vi "Zadanie11.vi"() -> ()   [LabVIEW 2020]
doc: "Project of sound reciving program, made by Rados³aw Bielak."
uses:
  <vilib>/sound2/lvsound2.llb/Sound Data Format.ctl
  Ctr4.ctl
  Ctr3.ctl
  datacons.ctl
  <vilib>/sound2/lvsound2.llb/Sound Input Task ID.ctl
  <vilib>/sound2/lvsound2.llb/Sampling Mode.ctl
  <vilib>/sound2/lvsound2.llb/Sound Input Read (DBL).vi
  <vilib>/sound2/lvsound2.llb/Sound File Write Open.vi
  <vilib>/sound2/lvsound2.llb/Sound File Write (DBL).vi
  <vilib>/measure/maspectr.llb/FFT Power Spectrum and PSD for N Chan.vi
  <vilib>/measure/NI_MAPro.lvlib
panel:
  in  "File Path":path
  in  "Sound Format":T1={"sample rate (S/s)"=22050.0, "number of channels"=2, "bits per sample"=16}
  in  "Sample Rate":i32=10000
  in  "Exit":bool
  in  "Play":bool
  in  "Tab Control":enum32{"Time Signal", "Power Spectrum"}(tab)
  out "Time Signal":waveform(dbl)[](graph)
  out "Power Spectrum":cluster{"f0":dbl, "df":dbl, "magnitude":dbl[]}[](graph)
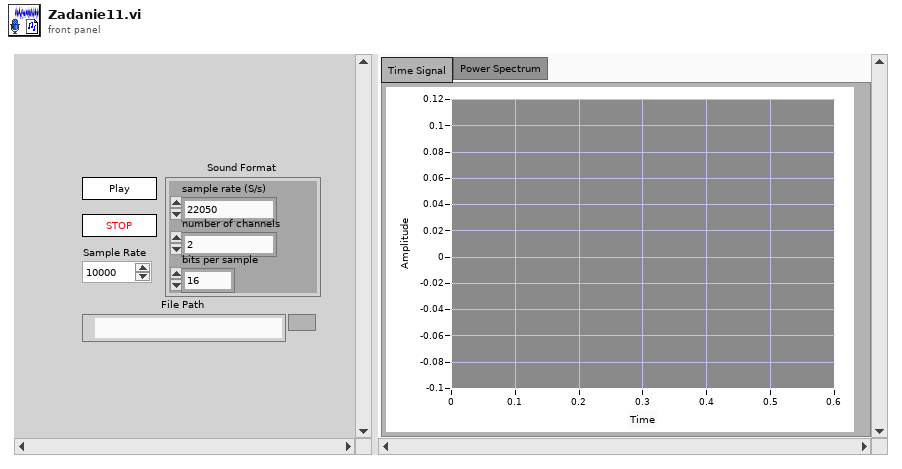
[diagram p1: front panel]
types:
  T1 = typedef "Sound Data Format.ctl" = cluster{"sample rate (S/s)":dbl, "number of channels":i32, "bits per sample":i32}
  T2 = typedef "Ctr4.ctl" = cluster{"Enum":T3, "data":variant}
  T3 = typedef "Ctr3.ctl" = enum16{"time", "spectrum"}
  T4 = typedef "datacons.ctl" = cluster{"Play":bool, "number of samples/ch":i32, "sound format":T1}
  T5 = typedef "Sound File Refnum.ctl" = refnum<file>
  T6 = typedef "Sound Input Task ID.ctl" = u32
  T7 = typedef "Sampling Mode.ctl" = i32
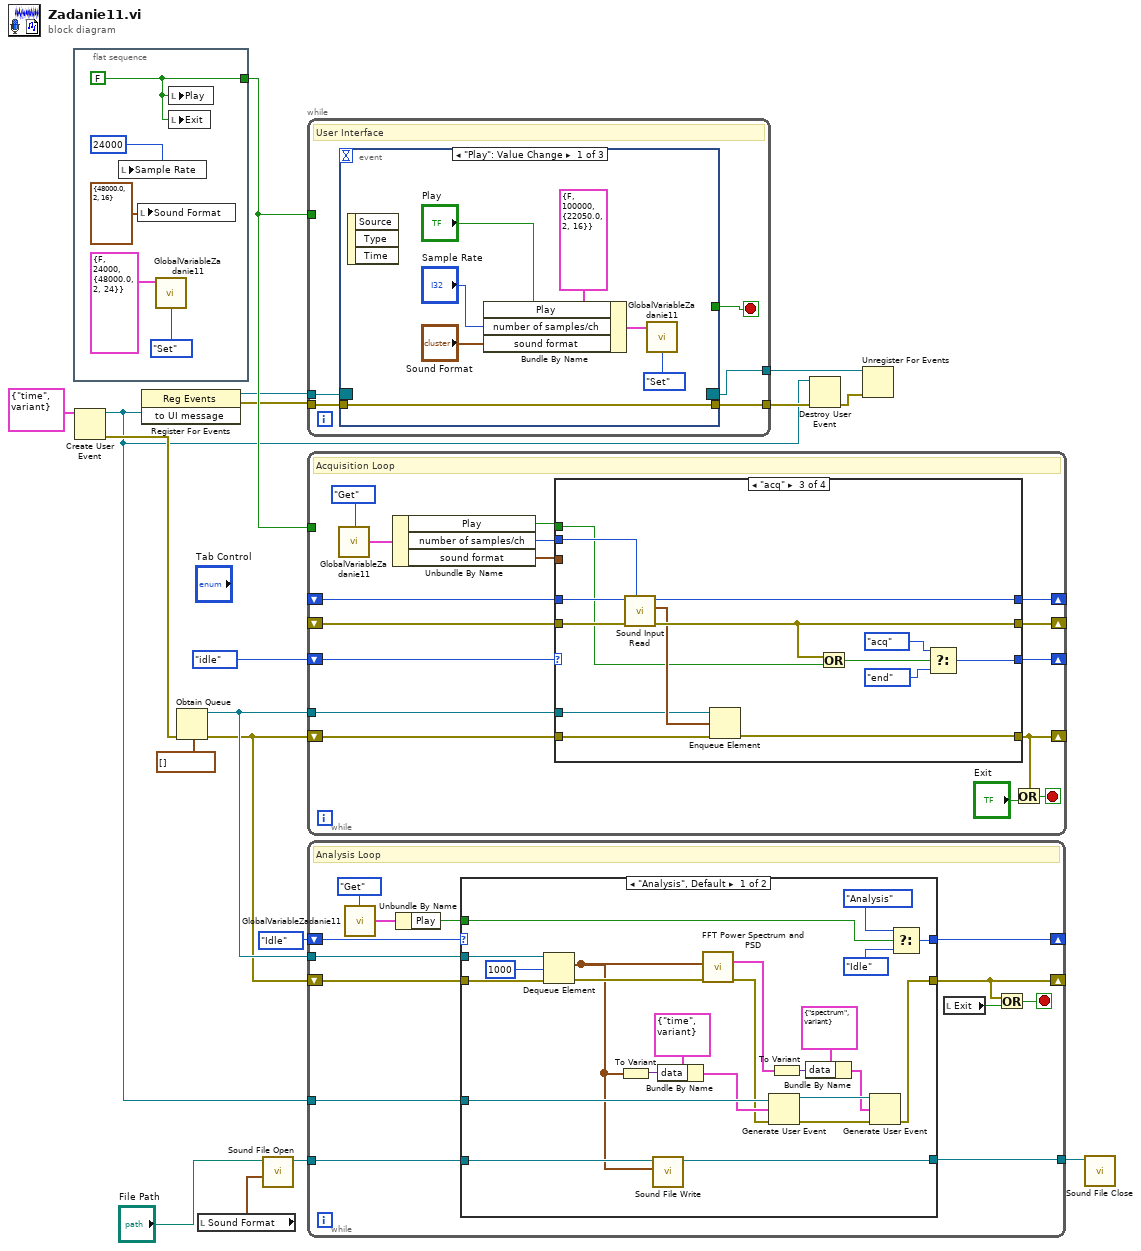
[diagram p0: block diagram]
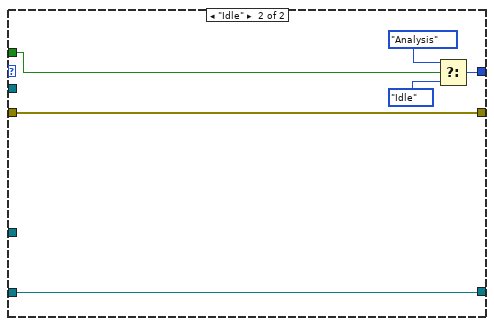
[diagram p2: hidden frame]
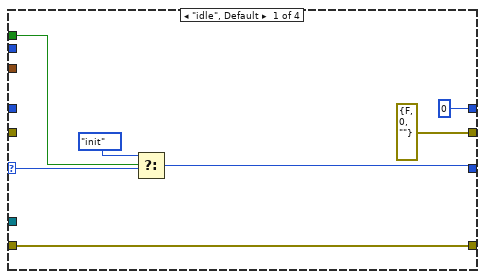
[diagram p3: hidden frame]
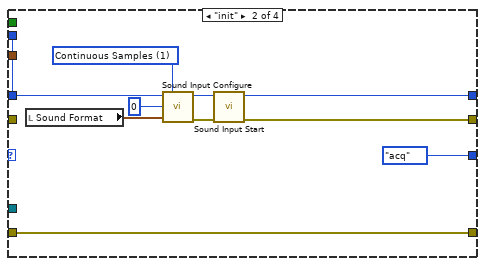
[diagram p4: hidden frame]
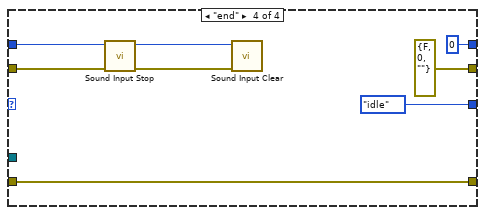
[diagram p5: hidden frame]
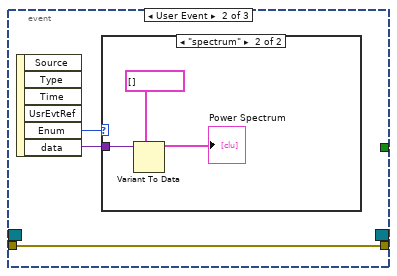
[diagram p6: hidden frame]
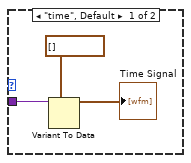
[diagram p7: hidden frame]
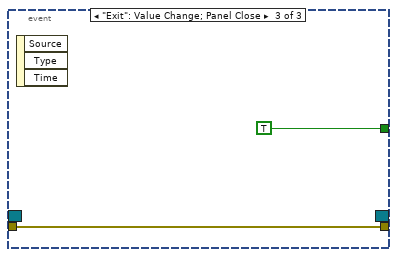
[diagram p8: hidden frame]
diagram:
  n1 = flat-sequence {
    tunnel: [w21] -> w18
    frame #0 {
      w21 = FALSE
      n2 = local write "Sample Rate"(24000) -> ()
      n3 = local write "Sound Format"(T1 {"sample rate (S/s)"=48000.0, "number of channels"=2, "bits per sample"=16} ("sound format")) -> ()
      n4 = call "GlobalVariableZadanie11.vi"("Action"=enum16{"Set", "Get"}."Set", "input"=T4 {"Play"=FALSE, "number of samples/ch"=24000, "sound format"={"sample rate (S/s)"=48000.0, "number of channels"=2, "bits per sample"=24}} ("cluster")) -> ()  [unwired: 9 in, 1 out]
      n5 = local write "Play"(w21) -> ()
      n6 = local write "Exit"(w21) -> ()
    }
  }
  n7 = Create User Event(user event datatype=T2 {"Enum"=enum."time", "data"=variant} ("to UI message")) -> (user event=w5:refnum<user-event>, error out=w13:errorcluster)  [unwired: 1 in]
  n8 = register-events(w5) -> (reference out=w9:refnum<event-registration>, error out=w8:errorcluster)  [unwired: 2 in]
  n9 = Obtain Queue(element data type=waveform(dbl)[] [] ("data"), error in (no error)=w13) -> (queue out=w16:refnum<queue>, error out=w10:errorcluster)  [unwired: 3 in, 1 out]
  n10 = local read "Sound Format"() -> (w4:T1)
  n11 = call-poly <vilib>:"Sound File Open.vi"("sound format"=w4, "path"="File Path") -> ("sound file refnum"=w3:T5)  [unwired: 8 in, 1 out]
  n12 = while "User Interface" {
    tunnel: w18 -> [_]
    tunnel: [w27] -> w12
    tunnel: w9 -> [w26]
    tunnel: w8 -> [w25]
    tunnel: [w24] -> w7
    stop <- w28 stop-if-true
    # "User Interface"
    n13 = event shown="[0] \"Play\": Value Change" {
      selector: w26 -> [_ _ _]
      dyn-events: [_ _ _] -> w27
      timeout: _ -> [_ _ _]
      tunnel: [_ _ TRUE] -> w28
      tunnel: w25 -> [w29 w36 w45]
      tunnel: [w29 w36 w45] -> w24
      event "Play": Value Change {
        n14 = event-data() -> ()  [unwired: 1 in, 3 out]
        n15 = Bundle By Name(cluster=T4 {"Play"=FALSE, "number of samples/ch"=100000, "sound format"={"sample rate (S/s)"=22050.0, "number of channels"=2, "bits per sample"=16}}, "Play"="Play", "number of samples/ch"="Sample Rate", "sound format"="Sound Format") -> (w31:T4)
        n16 = call "GlobalVariableZadanie11.vi"("Action"=enum16{"Set", "Get"}."Set", "input"=w31) -> ()  [unwired: 9 in, 1 out]
      }
      event User Event {
        n17 = event-data() -> ("Enum"=w38:T3, "data"=w37:variant)  [unwired: 1 in, 4 out]
        n18 = case shown="\"spectrum\"" w38 {
          tunnel: w37 -> [w41 w44]
          frame "time", Default {
            n19 = Variant To Data(type=waveform(dbl)[] [] ("element"), Variant=w41) -> (data=→"Time Signal":waveform(dbl)[])  [unwired: 1 in, 1 out]
          }
          frame "spectrum" {
            n20 = Variant To Data(type=cluster{"f0":dbl, "df":dbl, "magnitude":dbl[]}[] [] ("Power Spectrum / PSD"), Variant=w44) -> (data=→"Power Spectrum":cluster{"f0":dbl, "df":dbl, "magnitude":dbl[]}[])  [unwired: 1 in, 1 out]
          }
        }
      }
      event "Exit": Value Change; Panel Close {
        n21 = event-data() -> ()  [unwired: 1 in, 3 out]
      }
    }
  }
  n22 = while {
    tunnel: [w63] -> _
    tunnel: w18 -> [w63]
    shift-right: [w57] -> _
    shift-left: enum16{"idle", "init", "acq", "end"}."idle" -> [w58]
    shift-right: [w53] -> _
    shift-left: w10 -> [w56]
    shift-right: [w51] -> _
    shift-left: _ -> [w50]
    shift-right: [w49] -> _
    shift-left: _ -> [w48]
    tunnel: w16 -> [w47]
    stop <- w55 stop-if-true
    # "Acquisition Loop"
    n23 = call "GlobalVariableZadanie11.vi"("Action"=enum16{"Set", "Get"}."Get") -> ("output"=w61:T4)  [unwired: 10 in]
    n24 = Unbundle By Name(w61) -> ("Play"=w60:bool, "number of samples/ch"=w52:i32, "sound format"=w59:T1)
    n25 = case shown="\"acq\"" w58 {
      selector: w58 -> [w65 _ _ _]
      tunnel: [T6 0 ("task ID out") w76 w91 T6 0 ("task ID out")] -> w51
      tunnel: [errorcluster {"status"=FALSE, "code"=0, "source"=""} ("error out") w75 w90 errorcluster {"status"=FALSE, "code"=0, "source"=""} ("error out")] -> w49
      tunnel: w59 -> [_ _ _ _]
      tunnel: w50 -> [_ _ w84 w97]
      tunnel: w52 -> [_ w74 w85 _]
      tunnel: w60 -> [w67 _ w81 _]
      tunnel: w47 -> [_ _ w88 _]
      tunnel: w56 -> [w64 w72 w87 w95]
      tunnel: [w66 enum16{"idle", "init", "acq", "end"}."acq" w86 enum16{"idle", "init", "acq", "end"}."idle"] -> w57
      tunnel: [w64 w72 w82 w95] -> w53
      tunnel: w48 -> [_ _ w83 w96]
      frame "idle", Default {
        n26 = Select(t=enum16{"idle", "init", "acq", "end"}."init", s=w67, f=w65) -> (s? t:f=w66:enum16{"idle", "init", "acq", "end"})
      }
      frame "init" {
        w77 = T7 1 items=["Finite Samples", "Continuous Samples"] ("sample mode")
        n27 = local read "Sound Format"() -> (w71:T1)
        n28 = call <vilib>:"Sound Input Configure.vi"("number of samples/ch"=w74, "sample mode"=w77, "sound format"=w71, "device ID"=u32 0) -> ("error out"=w80:errorcluster, "task ID"=w79:T6)  [unwired: 6 in]
        n29 = call <vilib>:"Sound Input Start.vi"("error in (no error)"=w80, "task ID"=w79) -> ("error out"=w75:errorcluster, "task ID out"=w76:T6)  [unwired: 8 in]
      }
      frame "acq" {
        n30 = call-poly <vilib>:"Sound Input Read.vi"("number of samples/ch"=w85, "error in (no error)"=w83, "task ID"=w84) -> ("error out"=w90:errorcluster, "data"=w89:waveform(dbl)[], "task ID out"=w91:T6)  [unwired: 6 in]
        n31 = Enqueue Element(queue=w88, element=w89, error in (no error)=w87) -> (error out=w82:errorcluster)  [unwired: 1 in, 2 out]
        n32 = Or(x=w90, y=w81) -> (x .or. y?=w94:bool)
        n33 = Select(t=enum16{"idle", "init", "acq", "end"}."acq", s=w94, f=enum16{"idle", "init", "acq", "end"}."end") -> (s? t:f=w86:enum16{"idle", "init", "acq", "end"})
      }
      frame "end" {
        n34 = call <vilib>:"Sound Input Stop.vi"("error in (no error)"=w96, "task ID"=w97) -> ("error out"=w102:errorcluster, "task ID out"=w101:T6)  [unwired: 8 in]
        n35 = call <vilib>:"Sound Input Clear.vi"("error in (no error)"=w102, "task ID"=w101) -> ()  [unwired: 9 in, 1 out]
      }
    }
    n36 = Or(x=w53, y="Exit") -> (x .or. y?=w55:bool)
  }
  n37 = while {
    tunnel: w16 -> [w110]
    shift-right: [w111] -> _
    shift-left: enum16{"Analysis", "Idle"}."Idle" -> [w113]
    shift-right: [w106] -> _
    shift-left: w10 -> [w109]
    tunnel: w5 -> [w108]
    tunnel: w3 -> [w104]
    tunnel: [w103] -> w2
    stop <- w107 stop-if-true
    # "Analysis Loop"
    n38 = call "GlobalVariableZadanie11.vi"("Action"=enum16{"Set", "Get"}."Get") -> ("output"=w114:T4)  [unwired: 10 in]
    n39 = Unbundle By Name(w114) -> ("Play"=w112:bool)
    n40 = case shown="\"Analysis\", Default" w113 {
      tunnel: w112 -> [w138 w142]
      tunnel: [w136 w143] -> w111
      tunnel: w110 -> [w134 _]
      tunnel: w109 -> [w133 w144]
      tunnel: w108 -> [w128 _]
      tunnel: [w119 w144] -> w106
      tunnel: w104 -> [w118 w139]
      tunnel: [w117 w139] -> w103
      frame "Analysis", Default {
        n41 = Dequeue Element(queue=w134, timeout in ms (-1)=1000, error in (no error)=w133) -> (element=w116:waveform(dbl)[], error out=w131:errorcluster)  [unwired: 2 out]
        n42 = To Variant(anything=w116) -> (Variant=w130:variant)
        n43 = call-poly <vilib>:"Sound File Write.vi"("data"=w116, "sound file refnum"=w118) -> ("sound file refnum out"=w117:T5)  [unwired: 8 in, 1 out]
        n44 = Bundle By Name(cluster=T2 {"Enum"=enum."time", "data"=variant} ("to UI message"), "data"=w130) -> (w127:T2)
        n45 = call-poly <vilib>:"FFT Power Spectrum and PSD.vi"("error in (no error)"=w131, "time signals"=w116) -> ("error out"=w126:errorcluster, "Power Spectrum / PSD"=w123:cluster{"f0":dbl, "df":dbl, "magnitude":dbl[]}[])  [unwired: 6 in, 2 out]
        n46 = Generate User Event(user event=w128, event data cluster=w127, error in=w126) -> (user event out=w125:refnum<user-event>, error out=w124:errorcluster)  [unwired: 1 in]
        n47 = To Variant(anything=w123) -> (Variant=w122:variant)
        n48 = Bundle By Name(cluster=T2 {"Enum"=enum."spectrum", "data"=variant} ("to UI message"), "data"=w122) -> (w120:T2)
        n49 = Generate User Event(user event=w125, event data cluster=w120, error in=w124) -> (error out=w119:errorcluster)  [unwired: 1 in, 1 out]
        n50 = Select(t=enum16{"Analysis", "Idle"}."Analysis", s=w138, f=enum16{"Analysis", "Idle"}."Idle") -> (s? t:f=w136:enum16{"Analysis", "Idle"})
      }
      frame "Idle" {
        n51 = Select(t=enum16{"Analysis", "Idle"}."Analysis", s=w142, f=enum16{"Analysis", "Idle"}."Idle") -> (s? t:f=w143:enum16{"Analysis", "Idle"})
      }
    }
    n52 = local read "Exit"() -> (w105:bool)
    n53 = Or(x=w106, y=w105) -> (x .or. y?=w107:bool)
  }
  n54 = Destroy User Event(user event=w5, error in=w7) -> (error out=w6:errorcluster)
  n55 = Unregister For Events(event registration refnum=w12, error in=w6) -> ()  [unwired: 1 out]
  n56 = call <vilib>:"Sound File Close.vi"("sound file refnum"=w2) -> ()  [unwired: 10 in, 1 out]
